vi "MDAQ_SaveCVFile.vi"(8 "error in":errorcluster, 10 "Control Cluster":T2 {"CV"."Temperature Array" scale=0.0..100.0}, 11 "Concurrent CV Arrays":T1) -> (0 "error out":errorcluster)   [LabVIEW 2021]
uses:
  GUI_Def.ctl
  Mode_Enum.ctl
  Array_Cluster.ctl
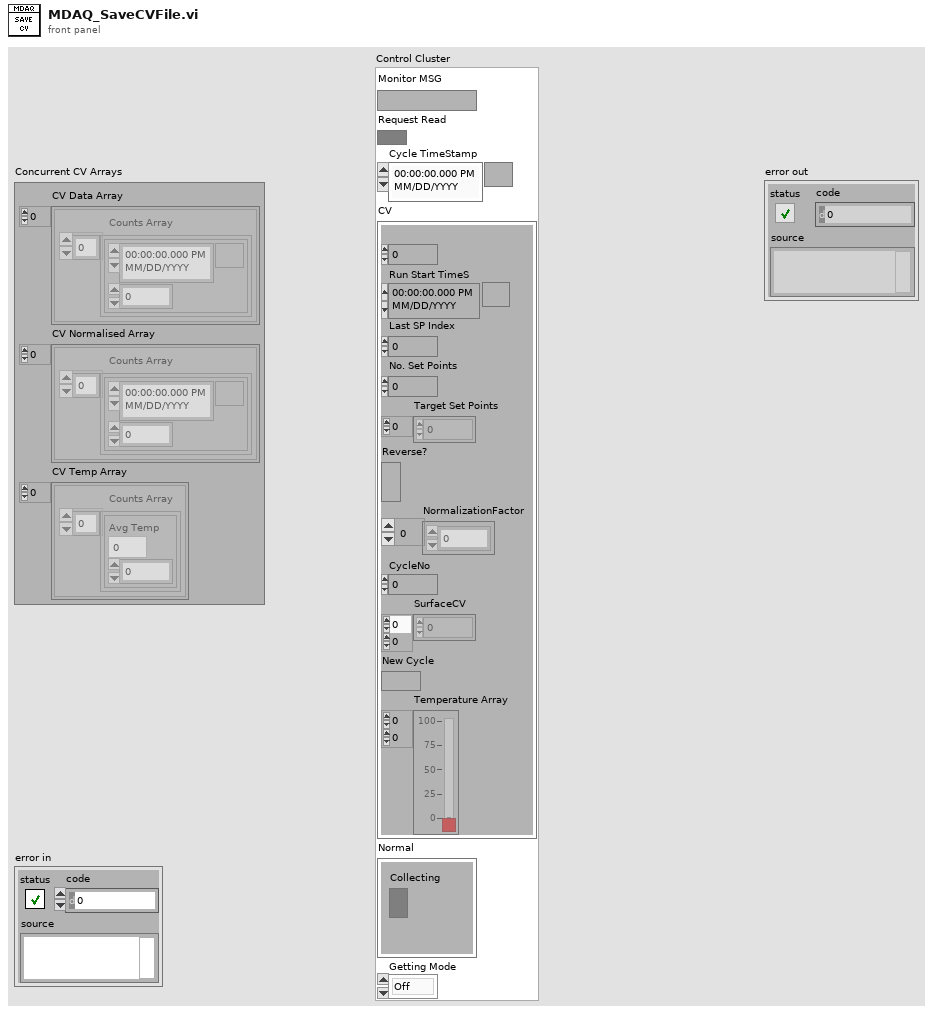
[diagram p1: front panel]
types:
  T1 = typedef "Array_Cluster.ctl" = cluster{"CV Data Array":cluster{"Counts Array":cluster{timestamp, i32}[]}[], "CV Normalised Array":cluster{"Counts Array":cluster{timestamp, dbl}[]}[], "CV Temp Array":cluster{"Counts Array":cluster{"Avg Temp":dbl, dbl}[]}[]}
  T2 = typedef "GUI_Def.ctl" = cluster{"Monitor MSG":string, "Request Read":bool, "Cycle TimeStamp":timestamp, "CV":cluster{"Set Point Index":u32, "Run Start TimeS":timestamp, "Last SP Index":u32, "No. Set Points":u32, "Target Set Points":i32[], "Reverse?":bool, "NormalizationFactor":i32[], "CycleNo":i32, "SurfaceCV":dbl[][], "New Cycle":bool, "Temperature Array":dbl[][]}, "Normal":cluster{"Collecting":bool}, "Getting Mode":T3}
  T3 = typedef "Mode_Enum.ctl" = enum16{"Off", "Normal", "CV+Temp", "CV"}
  T4 = enum16{"open", "replace", "create", "open or create", "replace or create", "replace or create with confirmation"}
  T5 = cluster{"Counts Array":cluster{timestamp, i32}[]}[]
  T6 = cluster{"Counts Array":cluster{timestamp, i32}[]}
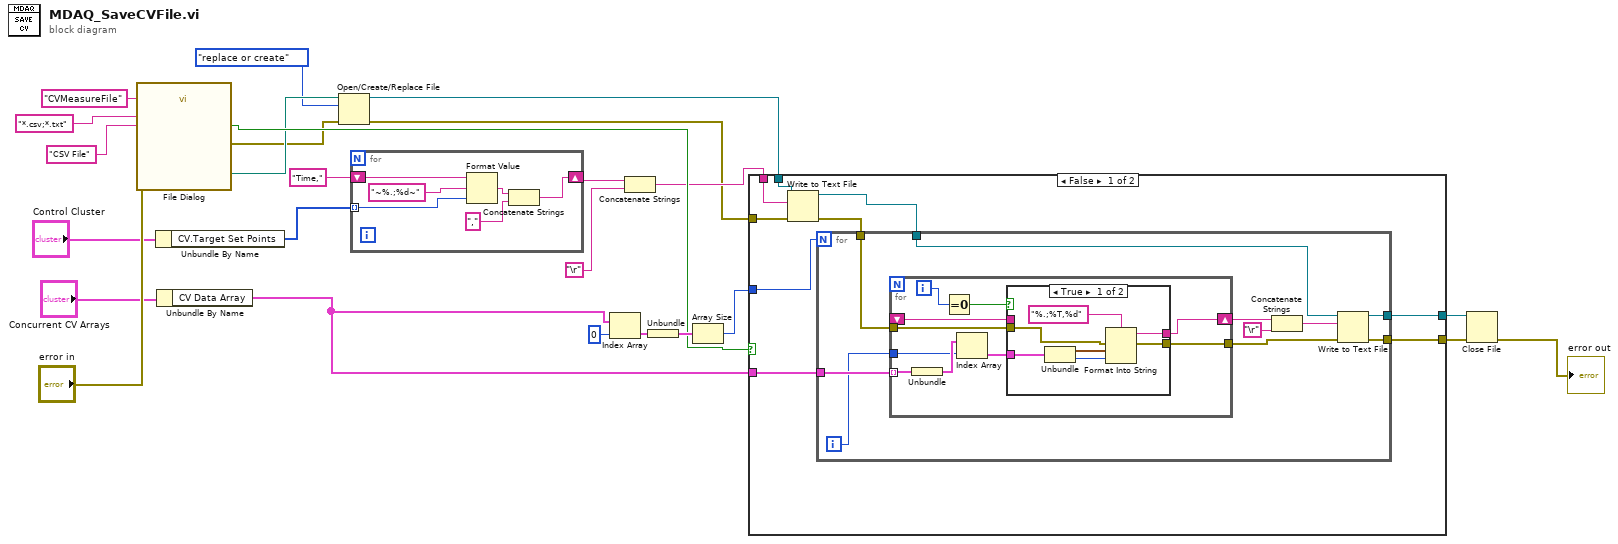
[diagram p0: block diagram]
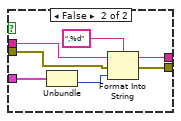
[diagram p2: hidden frame]
diagram:
  n1 = call "File Dialog"("default name"="CVMeasureFile", "error in"="error in", "pattern (all files)"="*.csv;*.txt", "pattern label"="CSV File") -> ("selected path"=w8:path, "cancelled"=w13:bool, "error out"=w6:errorcluster)  [unwired: 8 in, 1 out]
  n2 = Unbundle By Name("Control Cluster") -> ("CV.Target Set Points"=w21:i32[])
  n3 = Unbundle By Name("Concurrent CV Arrays") -> ("CV Data Array"=w1:T5)
  n4 = Open/Create/Replace File(file path (use dialog)=w8, error in=w6, operation (0:open)=T4."replace or create") -> (refnum out=w4:refnum<file>, error out=w5:errorcluster)  [unwired: 3 in, 1 out]
  n5 = for {
    tunnel: w21 -> [w30] mode=indexing
    shift-right: [w28] -> w19
    shift-left: "Time," ("text") -> [w31]
    n6 = Format Value(string ("")=w31, format string="~%.;%d~", value (0)=w30) -> (output string=w27:string)
    n7 = Concatenate Strings(w27, ",") -> (w28:string)
  }
  n8 = Index Array(array=w1, index=0) -> (element=w16:T6)
  n9 = Concatenate Strings(w19, "\r") -> (w12:string)
  n10 = Unbundle(w16) -> ("Counts Array"=w15:cluster{timestamp, i32}[])
  n11 = Array Size(array=w15) -> (size(s)=w14:i32)
  n12 = case shown="False" w13 {
    tunnel: w1 -> [w40 _]
    tunnel: w14 -> [w39 _]
    tunnel: [w38 w76] -> w10
    tunnel: w5 -> [w37 w76]
    tunnel: w12 -> [w36 _]
    tunnel: w4 -> [w35 w75]
    tunnel: [w32 w75] -> w11
    frame False {
      n13 = Write to Text File(file (use dialog)=w35, text=w36, error in=w37) -> (refnum out=w33:refnum<file>, error out=w34:errorcluster)  [unwired: 1 in, 1 out]
      n14 = for {
        N: w39 -> [_]
        tunnel: w40 -> [w50]
        tunnel: w34 -> [w49]
        tunnel: w33 -> [w44]
        tunnel: [w43] -> w38
        tunnel: [w42] -> w32
        i -> [w41]
        n15 = for {
          tunnel: w50 -> [w60] mode=indexing
          tunnel: w41 -> [w58]
          tunnel: w49 -> [w55]
          tunnel: [w54] -> w45
          shift-right: [w53] -> w48
          shift-left: _ -> [w52]
          i -> [w51]
          n16 = Unbundle(w60) -> ("Counts Array"=w59:cluster{timestamp, i32}[])
          n17 = Equal To 0?(x=w51) -> (x = 0?=w57:bool)
          n18 = Index Array(array=w59, index=w58) -> (element=w56:cluster{timestamp, i32})
          n19 = case shown="True" w57 {
            tunnel: w56 -> [w67 w74]
            tunnel: w55 -> [w63 w72]
            tunnel: [w62 w71] -> w54
            tunnel: [w61 w70] -> w53
            tunnel: w52 -> [_ w68]
            frame True {
              n20 = Unbundle(w67) -> (w65:timestamp, w64:i32)
              n21 = Format Into String(format string="%.;%T,%d", error in=w63, w65, w64) -> (resulting string=w61:string, error out=w62:errorcluster)  [unwired: 1 in]
            }
            frame False {
              n22 = Unbundle(w74) -> (w69:i32)  [unwired: 1 out]
              n23 = Format Into String(format string=",%d", initial string=w68, error in=w72, w69) -> (resulting string=w70:string, error out=w71:errorcluster)
            }
          }
        }
        n24 = Concatenate Strings(w48, "\r") -> (w46:string)
        n25 = Write to Text File(file (use dialog)=w44, text=w46, error in=w45) -> (refnum out=w42:refnum<file>, error out=w43:errorcluster)  [unwired: 1 in, 1 out]
      }
    }
    frame True {
    }
  }
  n26 = Close File(refnum=w11, error in=w10) -> (error out=→"error out":errorcluster)  [unwired: 1 out]
